vi "Dateiname mit Projektname Version GeraeteType SerienNummer und Zeitstempel.vi"(7 "Pfad":string, 10 "Extension in":string, 11 "File Name in":string) -> (3 "File Name":string)   [LabVIEW 2020, in "SysLog.lvlib"]
doc: "Hängt dem angegebenen Dateinamen einen Zeitstempel an, bei dem die Sonderzeichen Verzeichnis kompatibel ersetzt wurden + extension, Pfad vorangestellt ohne Filterung.\nStellt davor ProjektName, Version, GeräteType und SerienNummer\nriw 8.6.2018"
uses:
  SysLog.lvlib
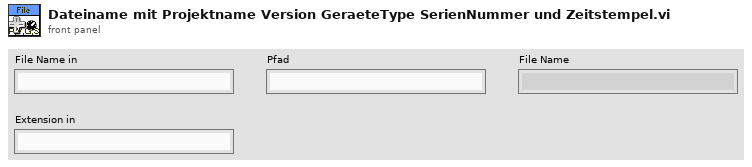
[diagram p1: front panel]
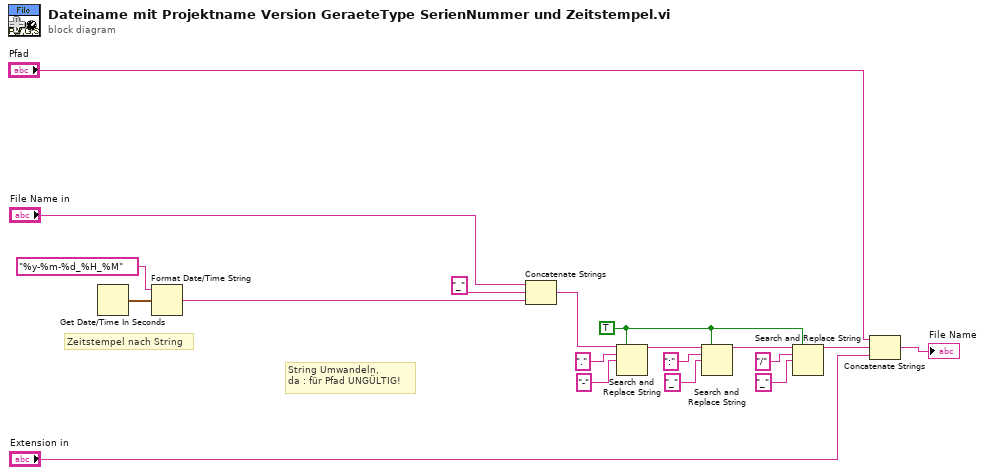
[diagram p0: block diagram]
diagram:
  w10 = TRUE ("Alle ersetzen? (F)")
  # "String Umwandeln, \nda : für Pfad UNGÜLTIG!"
  # "Zeitstempel nach String"
  n1 = Get Date/Time In Seconds() -> (seconds since 1Jan1904=w19:timestamp)
  n2 = Format Date/Time String(time format string (%c)="%y-%m-%d_%H_%M" ("Zeitformatierungs-String (%c)"), seconds (now)=w19) -> (date/time string=w7:string)  [unwired: 1 in]
  n3 = Concatenate Strings("File Name in", "_", w7) -> (w6:string)
  n4 = Search and Replace String(replace all?=w10, input string=w6, search string="." ("Such-String"), replace string="-" ("String ersetzen(\"\")")) -> (result string=w16:string)  [unwired: 4 in, 3 out]
  n5 = Search and Replace String(replace all?=w10, input string=w16, search string=":" ("Such-String"), replace string="_" ("String ersetzen(\"\")")) -> (result string=w11:string)  [unwired: 4 in, 3 out]
  n6 = Search and Replace String(replace all?=w10, input string=w11, search string="/" ("Such-String"), replace string="_" ("String ersetzen(\"\")")) -> (result string=w5:string)  [unwired: 4 in, 3 out]
  n7 = Concatenate Strings("Pfad", w5, "Extension in") -> (→"File Name":string)
